vi "Lee DB.vi"(8 "error in (no error)":errorcluster, 11 "Class 2 in":refnum<class "Class 2.lvclass">) -> (0 "error out":errorcluster, 3 "Class 2 out":refnum<class "Class 2.lvclass">)   [LabVIEW 2019, in "Class 2.lvclass"]
uses:
  Class 2.lvclass
  Class 2.lvclass/Class 2.ctl
  <vilib>/addons/database/Connection.llb/DB Tools Open Connec (Path).vi
  <vilib>/addons/database/_DB Variant To Data/Database Variant To Data.xnode
  <vilib>/addons/database/NI_Database_API.lvlib
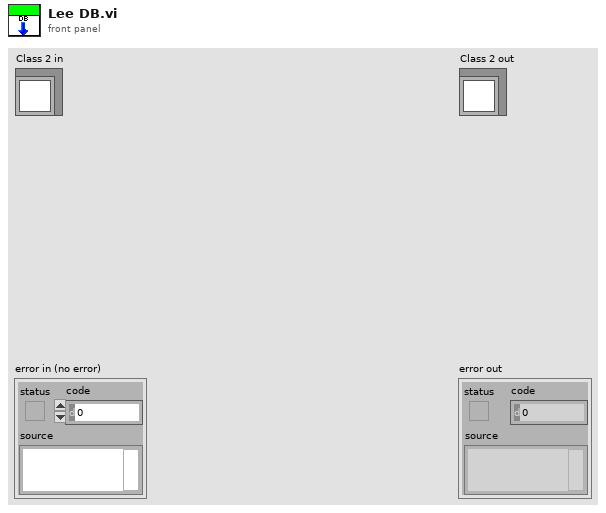
[diagram p1: front panel]
types:
  T1 = typedef "NI_Database_API.lvlib/Conn ObjectReference.ctl" = refnum<k1>
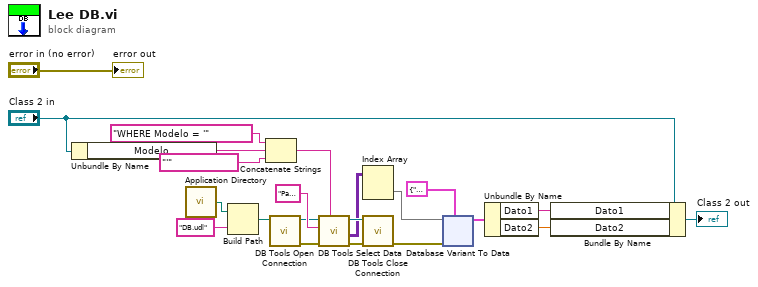
[diagram p0: block diagram]
diagram:
  n1 = Unbundle By Name("Class 2 in") -> ("Modelo"=w4:string)
  n2 = call <vilib>:"Application Directory.vi"() -> ("Application Directory"=w12:path)
  n3 = Build Path(base path=w12, name or relative path="DB.udl") -> (appended path=w10:path)
  n4 = Concatenate Strings("WHERE Modelo = '" ("string"), w4, "'" ("string")) -> (w6:string)
  n5 = call-poly <vilib>:"DB Tools Open Connection.vi"("connection information"=w10) -> ("error out"=w14:errorcluster, "connection reference"=w13:T1)  [unwired: 7 in]
  n6 = call <vilib>:"DB Tools Select Data.vi"("condition"=w6, "error in (no error)"=w14, "table"="Parametros", "connection reference"=w13) -> ("error out"=w19:errorcluster, "data"=w16:variant[][], "connection reference out"=w17:T1)  [unwired: 2 in]
  n7 = Index Array(array=w16) -> (element=w15:variant[])  [unwired: 2 in]
  n8 = call <vilib>:"DB Tools Close Connection.vi"("error in (no error)"=w19, "connection reference"=w17) -> ("error out"=w9:errorcluster)  [unwired: 5 in]
  n9 = xnode "Database Variant To Data"("database variant"=w15, "error in (no error)"=w9, "type"=cluster{"Dato1":string, "Dato2":dbl} {"Dato1"="", "Dato2"=0.0} ("Parametros")) -> ("data"=w3:cluster{"Dato1":string, "Dato2":dbl})  [unwired: 1 out]
  n10 = Unbundle By Name(w3) -> ("Dato1"=w2:string, "Dato2"=w1:dbl)
  n11 = Bundle By Name(cluster="Class 2 in", "Dato1"=w2, "Dato2"=w1) -> (→"Class 2 out":refnum<class "Class 2.lvclass">)
  "error out" <- "error in (no error)"
